vi "GEOM_CorrectByRotation.vi"(9 "Amplifiers":T1[](array[typedef]) {"fliped" items=["none", "horizontal", "vertical"]; "type" items=["LL", "LR", "UL", "UR"]}, 10 "rotate ROIs?":bool=TRUE) -> (1 "rotated amps":T1[](array[typedef]) {"fliped" items=["none", "horizontal", "vertical"]; "type" items=["LL", "LR", "UL", "UR"]}, 2 "any rotated?":bool)   [LabVIEW 2016]
uses:
  GEOM_Amplifier.ctl
  GEOM_AmpType.ctl
  GEOM_ROI.ctl
  GEOM_Coords.ctl
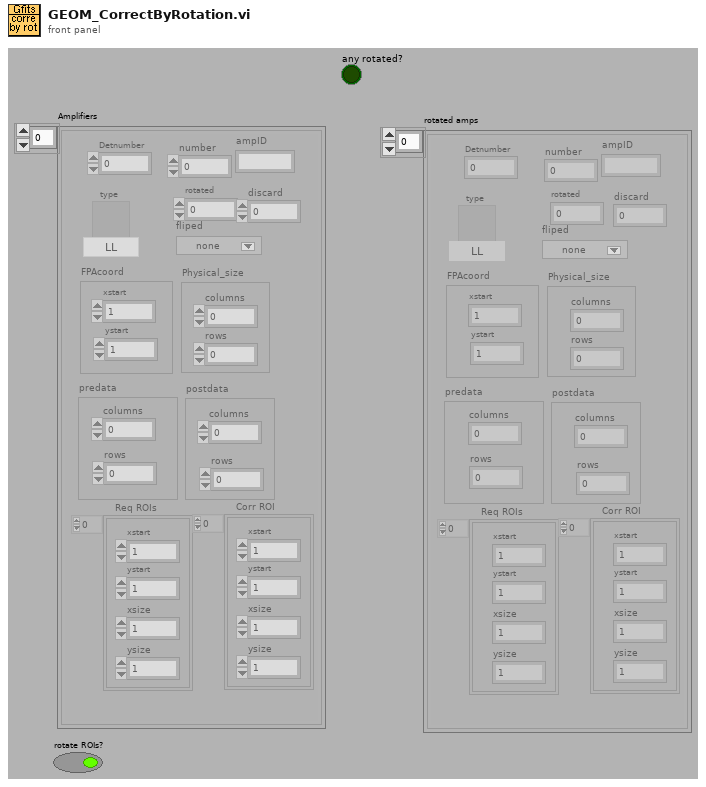
[diagram p1: front panel]
types:
  T1 = typedef "GEOM_Amplifier.ctl" = cluster{"number":i32, "type":T2, "rotated":i16, "fliped":u16, "FPAcoord":cluster{"xstart":i32, "ystart":i32}, "Physical_size":cluster{"columns":i32, "rows":i32}, "predata":cluster{"columns":i32, "rows":i32}, "postdata":cluster{"columns":i32, "rows":i32}, "Req ROIs":T3, "Corr ROI":T3, "Detnumber":i32, "ampID":string, "discard":i32}
  T2 = typedef "GEOM_AmpType.ctl" = u16
  T3 = typedef "GEOM_ROI.ctl" = T4[]
  T4 = typedef "GEOM_Coords.ctl" = cluster{"xstart":u32, "ystart":u32, "xsize":u32, "ysize":u32}
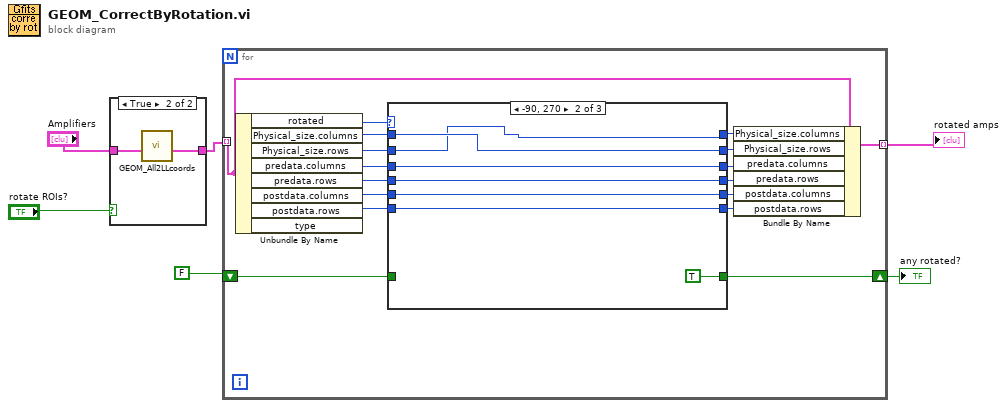
[diagram p0: block diagram]
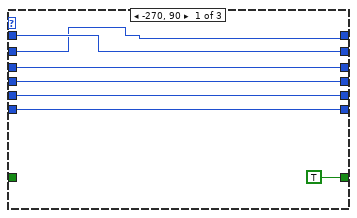
[diagram p3: hidden frame]
diagram:
  n1 = case shown="True" "rotate ROIs?" {
    tunnel: "Amplifiers" -> [w7 w9]
    tunnel: [w7 w8] -> w3
    frame False {
    }
    frame True {
      n2 = call "GEOM_All2LLcoords.vi"("Amplifiers"=w9) -> ("Amps with LL ROIs"=w8:T1[])  [unwired: 10 out]
    }
  }
  n3 = for {
    tunnel: w3 -> [w20] mode=indexing
    tunnel: [w24] -> w6 mode=indexing
    shift-right: [w10] -> w1
    shift-left: FALSE -> [w11]
    n4 = Unbundle By Name(w20) -> ("rotated"=w21:i16, "Physical_size.columns"=w26:i32, "Physical_size.rows"=w25:i32, "predata.columns"=w19:i32, "predata.rows"=w17:i32, "postdata.columns"=w15:i32, "postdata.rows"=w13:i32)  [unwired: 1 out]
    n5 = case shown="-90, 270" w21 {
      tunnel: w26 -> [w33 w40 w47]
      tunnel: w25 -> [w32 w39 w46]
      tunnel: [w32 w39 w47] -> w23
      tunnel: [w33 w40 w46] -> w22
      tunnel: [w30 w37 w45] -> w18
      tunnel: w19 -> [w30 w37 w45]
      tunnel: w17 -> [w29 w36 w44]
      tunnel: [w29 w36 w44] -> w16
      tunnel: w15 -> [w28 w35 w43]
      tunnel: [w28 w35 w43] -> w14
      tunnel: w13 -> [w27 w34 w42]
      tunnel: [w27 w34 w42] -> w12
      tunnel: w11 -> [_ _ w41]
      tunnel: [TRUE TRUE w41] -> w10
      frame -270, 90 {
      }
      frame -90, 270 {
      }
      frame 0, Default {
      }
    }
    n6 = Bundle By Name(cluster=w20, "Physical_size.columns"=w23, "Physical_size.rows"=w22, "predata.columns"=w18, "predata.rows"=w16, "postdata.columns"=w14, "postdata.rows"=w12) -> (w24:T1)
  }
  "rotated amps" <- w6
  "any rotated?" <- w1
